vi "RPi_I2C_BME280_Device_Intialize.vi"(0 "LINX Resource in":T1, 1 "I2C Channel (0)":u8, 2 "I2C Slave Address (0)":u8, 11 "error in (no error)":errorcluster) -> (4 "LINX Resource out":T1, 15 "error out":errorcluster)   [LabVIEW 2020]
doc: "Initializes the BME280 device for operation in 'Normal mode'.\n\nNormal mode: perpetual cycling of measurements and inactive periods.\n\nMIT License\nCopyright (c) 2021 Asper"
uses:
  <vilib>/MakerHub/LINX/Private/Type Defs/LINX Ref.ctl
  <vilib>/MakerHub/LINX/Private/Type Defs/Platform.ctl
  <vilib>/MakerHub/LINX/Private/Type Defs/Interface.ctl
  <vilib>/MakerHub/LINX/Private/Device/Type Defs/LINX Device Config.ctl
  <vilib>/MakerHub/LINX/Private/Device/Type Defs/TCP Config.ctl
  <vilib>/MakerHub/LINX/Private/Device/Type Defs/Channels.ctl
  <vilib>/MakerHub/LINX/Private/Local IO/LinxI2cWrite.vi
  <vilib>/MakerHub/LINX/Public/Utilities/Check Channel.vi
  <vilib>/MakerHub/LINX/Private/Local IO/Handle Errors.vi
  <vilib>/MakerHub/LINX/Private/Utilties/Generate Error.vi
  <vilib>/MakerHub/LINX/LMH-LINX.lvlib
  <vilib>/MakerHub/LINX/Private/Device/Device.lvlib
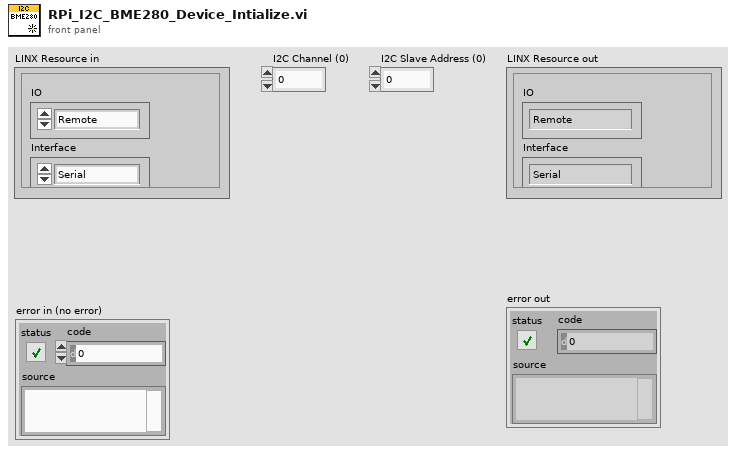
[diagram p1: front panel]
types:
  T1 = typedef "LMH-LINX.lvlib/LINX Ref.ctl" = cluster{"IO":T2, "Interface":T3, "LINX Device Config":T4}
  T2 = typedef "LMH-LINX.lvlib/Platform.ctl" = enum16{"Remote", "Local"}
  T3 = typedef "LMH-LINX.lvlib/Interface.ctl" = enum16{"Serial", "TCP"}
  T4 = typedef "LMH-LINX.lvlib/Device.lvlib/LINX Device Config.ctl" = cluster{"Interface":T3, "COM Port":refnum<visa-resource-name>, "TCP Configuration":T5, "Device Family":u8, "Device ID":u8, "Device Name":string, "TCP Ref":refnum<k5>, "Channels":T6}
  T5 = typedef "LMH-LINX.lvlib/Device.lvlib/TCP Config.ctl" = cluster{"IP Address":string, "Port":u16}
  T6 = typedef "LMH-LINX.lvlib/Channels.ctl" = cluster{"DI":u8[], "DO":u8[], "AI":u8[], "AO":u8[], "PWM":u8[], "QE":u8[], "UART":u8[], "I2C 2":u8[], "SPI":u8[], "CAN":u8[], "Servo":u8[], "AI Ref (V)":dbl, "AI Resolution (Bits)":u8, "AO Ref (V)":dbl, "AO Resolution (Bits)":u8}
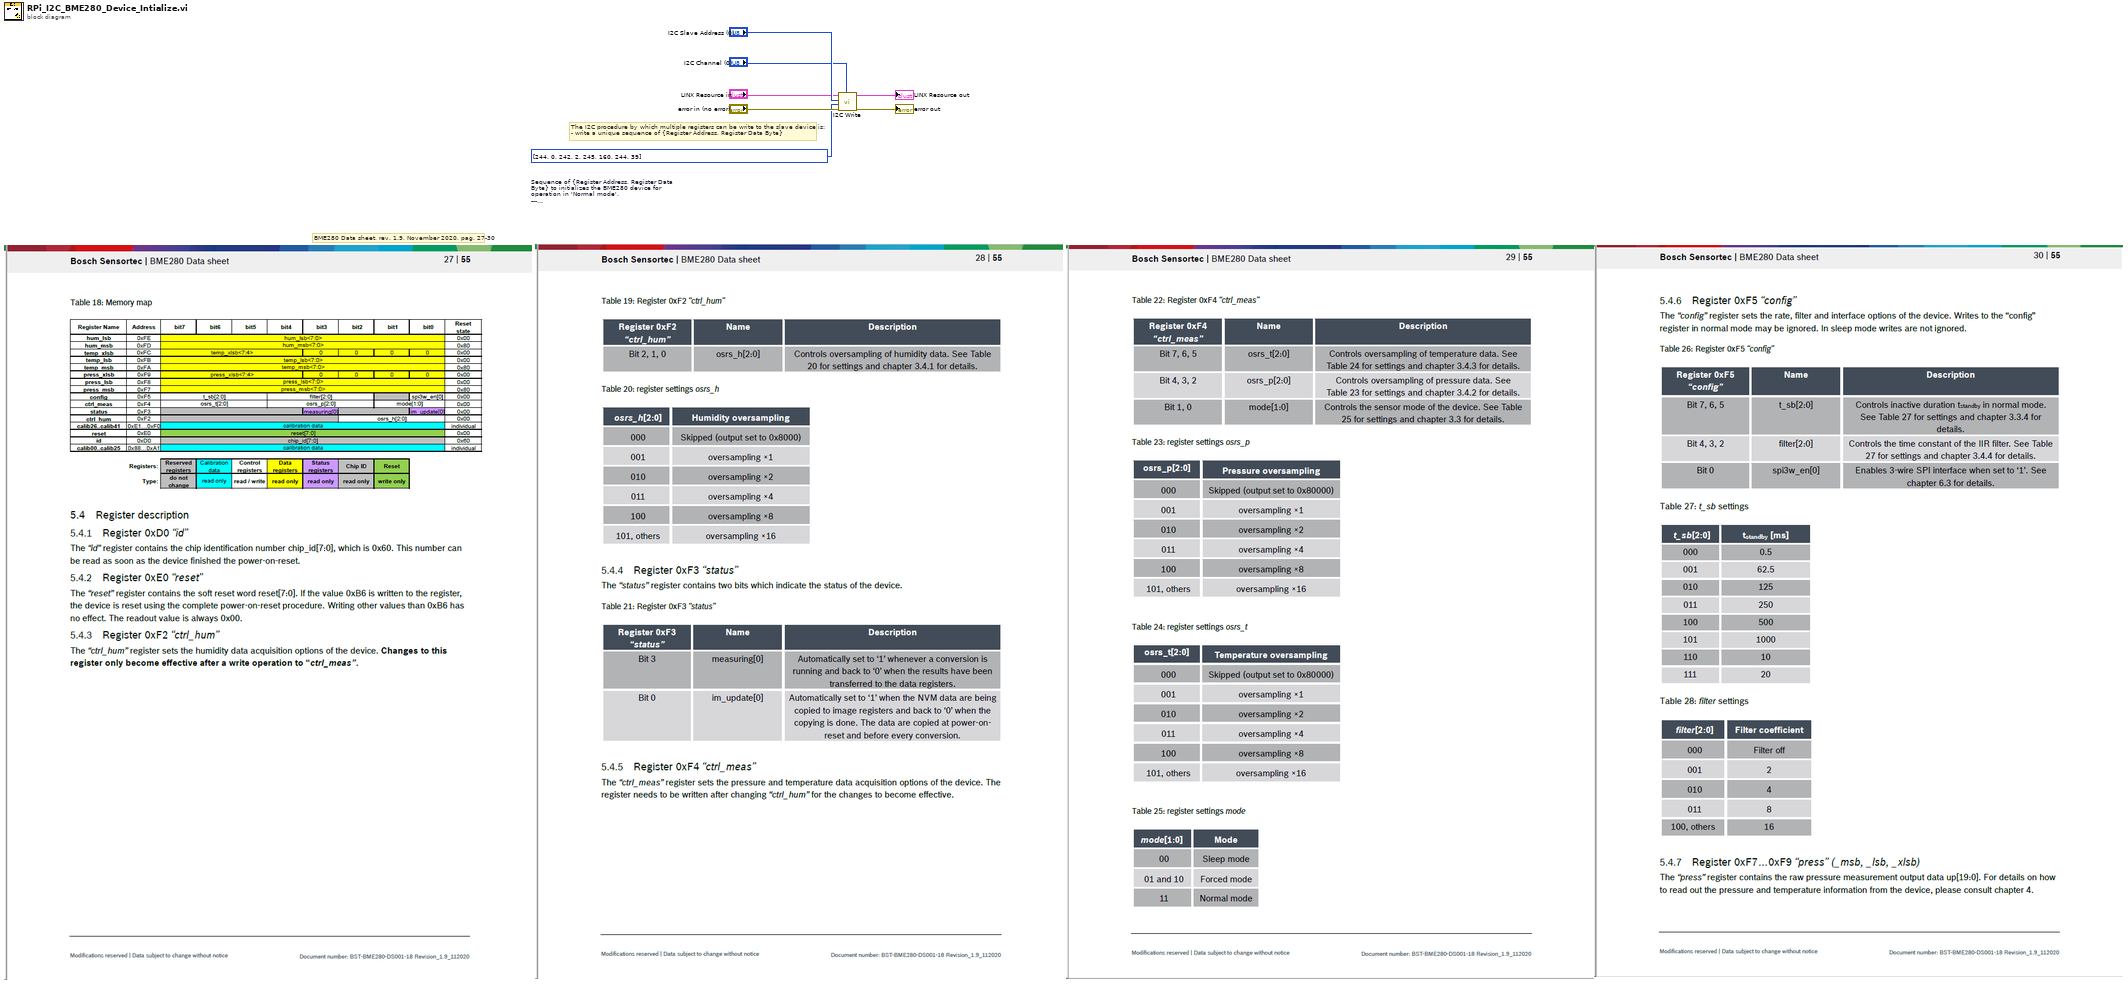
[diagram p0: block diagram]
diagram:
  w1 = u8[] [244, 0, 242, 2, 245, 160, 244, 39]  # Sequence of {Register Address, Register Data Byte} to initializes the BME280 device for operation in 'Normal mode'. --- xF4 - x00 Set Sleep mode  xF2 - x01 Set Humidity Oversampling xF5 -xA0 Set Tstandby 1000ms xF4 - x27 Set Temperature and Pressure Oversampling; Set 'Normal mode'
  # "BME280 Data sheet, rev. 1.9, November 2020, pag. 27-30"
  # "The I2C procedure by which multiple registers can be write to the slave device is:\n- write a unique sequence of {Register Address, Register Data Byte}"
  n1 = call <vilib>:"I2C Write.vi"("I2C Channel"="I2C Channel (0)", "Error In"="error in (no error)", "Data"=w1, "I2C Slave Address (0)"="I2C Slave Address (0)", "LINX Resource"="LINX Resource in") -> ("Error Out"=→"error out":errorcluster, "LINX Resource"=→"LINX Resource out":T1)  [unwired: 5 in]
